vi "Pid_v15.vi"() -> ()   [LabVIEW 2020]
panel:
  out "u - Comanda":dbl(graph)=49.999877814419186
  out "y - Iesirea":dbl(slide)=49.99941110945184 scale=40.0..60.0
  in  "stop":bool
  out "y":dbl=49.99941110945184
  out "u - Comanda":dbl(slide)=49.999877814419186 scale=40.0..60.0
  out "u,y,r":cluster{"r-Set point":dbl, dbl, dbl}(graph)={"r-Set point"=49.99941110945184, 50.0, 49.999877814419186}
  in  "Kd":dbl(slide)=0.1111111111111111 scale=0.0..0.5
  in  "Kp":dbl(slide)=0.3508771929824561 scale=0.0..2.5
  in  "Ki":dbl(slide)=0.8888888888888888 scale=0.0..2.0
  in  "r - Set point":dbl(slide)=50.0 scale=40.0..60.0
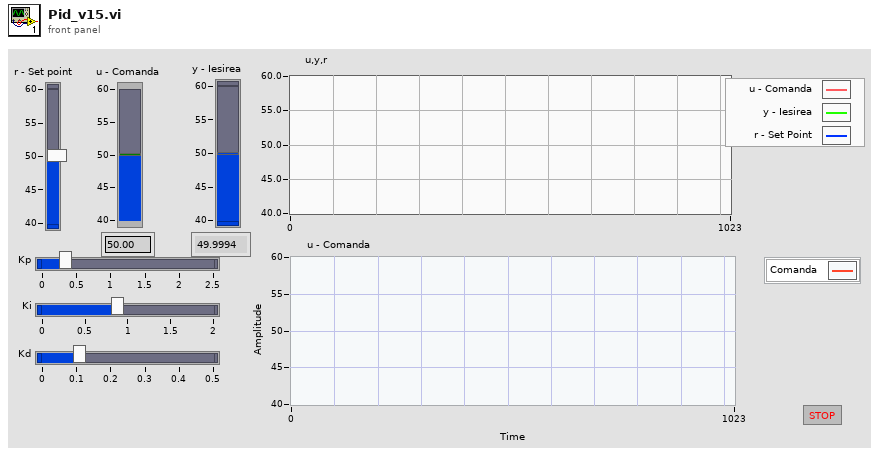
[diagram p1: front panel]
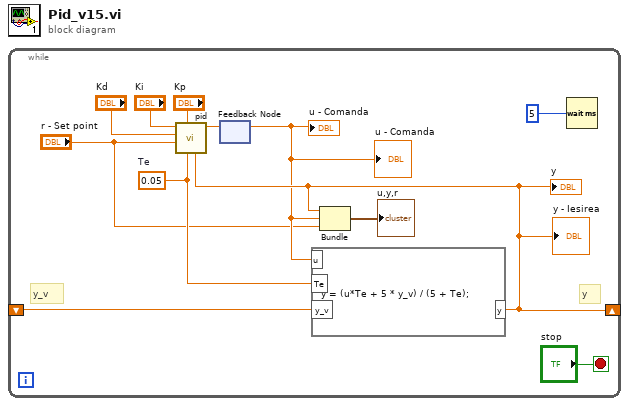
[diagram p0: block diagram]
diagram:
  n1 = while {
    shift-right: [w4] -> _
    shift-left: _ -> [w11]
    stop <- "stop" stop-if-true
    w6 = 0.05  # Te
    # "y_v"
    # "y"
    n2 = feedback #1() -> (w3:dbl)  [unwired: 1 in]
    "u - Comanda" <- w3
    "u - Comanda" <- w3
    n3 = formula code="y = (u*Te + 5 * y_v) / (5 + Te);"("y_v"=w11, "u"=w3, "Te"=w6) -> ("y"=w4:dbl)
    "y" <- w4
    "y - Iesirea" <- w4
    n4 = call "pid.vi"("y"=w4, "Te"=w6, "Kp"="Kp", "r - Set point"="r - Set point", "Kd"="Kd", "Ki"="Ki") -> ("u"=w5:dbl)  [unwired: 5 in]
    n5 = feedback-in #1(w5) -> ()
    n6 = Bundle("y"=w4, "u"=w3, "r - Set point"="r - Set point") -> (→"u,y,r":cluster{"y":dbl, "u":dbl, "r - Set point":dbl})  [unwired: 1 in]
    n7 = Wait (ms)(milliseconds to wait=u32 5) -> ()  [unwired: 1 out]
  }
